vi "Get gRPC Package Name.vi"(8 "error in (no error)":errorcluster, 11 "Pacakge ref in":u64) -> (0 "error out":errorcluster, 2 "Package Name":string, 3 "Package ref out":u64)   [LabVIEW 2019, in "gRPC Template Creation Utility.lvlib"]
uses:
  gRPC Template Creation Utility.lvlib
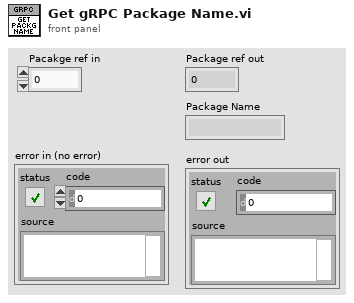
[diagram p1: front panel]
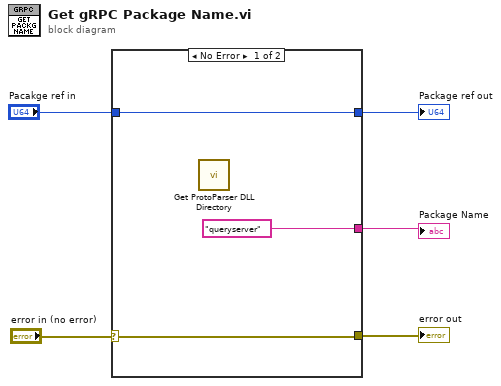
[diagram p0: block diagram]
diagram:
  n1 = case shown="No Error" "error in (no error)" {
    selector: "error in (no error)" -> [w7 w9]
    tunnel: "Pacakge ref in" -> [w8 w10]
    tunnel: [w7 w9] -> w3
    tunnel: [w8 w10] -> w2
    tunnel: ["queryserver" ("Package Name") _] -> w1
    frame No Error {
      n2 = call "Get ProtoParser DLL Directory.vi"() -> ()  [unwired: 1 out]
    }
    frame Error {
    }
  }
  "Package Name" <- w1
  "error out" <- w3
  "Package ref out" <- w2
